vi "Module Support.vi"() -> (6 "ge_DAQManDefinitions":T1)   [LabVIEW 2012]
uses:
  Controls/DAQMan Definitions.ctl
  Custom Ctrls/ge_MeasType.ctl
  Controls/Timing Engine Support.ctl
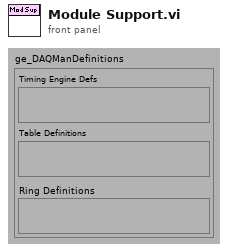
[diagram p1: front panel]
types:
  T1 = typedef "DAQMan Definitions.ctl" = cluster{"Timing Engine Defs":variant, "Table Definitions":variant, "Ring Definitions":variant}
  T2 = typedef "ge_MeasType.ctl" = enum16{"Voltage", "Frequency", "Tachometer", "Dynamic", "Thermocouple", "RTD", "Strain", "Current", "Resistance"}
  T3 = typedef "Timing Engine Support.ctl" = enum16{"HS Mod", "LS Mod", "Either"}
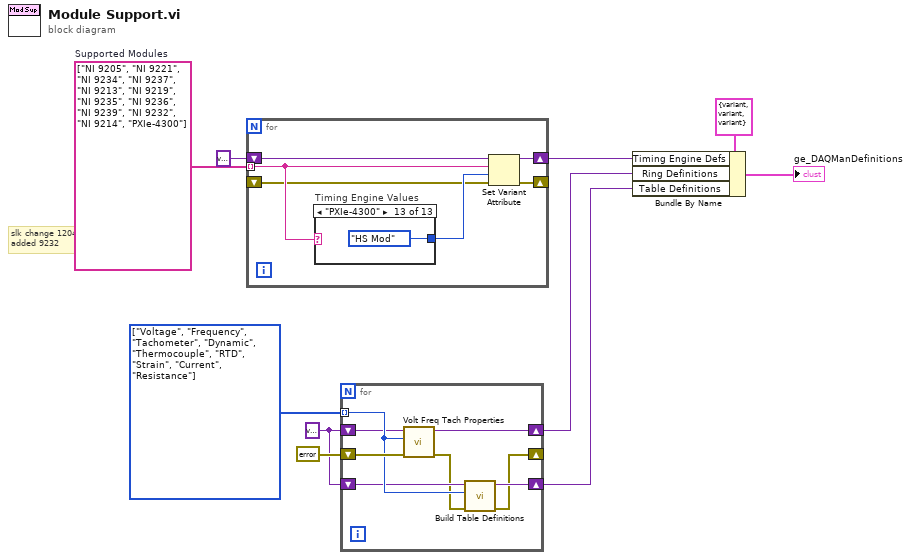
[diagram p0: block diagram]
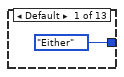
[diagram p2: hidden frame]
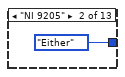
[diagram p3: hidden frame]
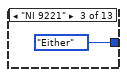
[diagram p4: hidden frame]
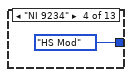
[diagram p5: hidden frame]
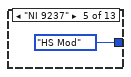
[diagram p6: hidden frame]
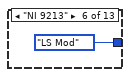
[diagram p7: hidden frame]
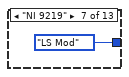
[diagram p8: hidden frame]
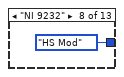
[diagram p9: hidden frame]
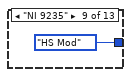
[diagram p10: hidden frame]
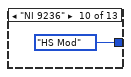
[diagram p11: hidden frame]
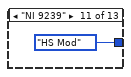
[diagram p12: hidden frame]
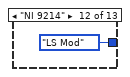
[diagram p13: hidden frame]
diagram:
  w7 = string[] ["NI 9205", "NI 9221", "NI 9234", "NI 9237", "NI 9213", "NI 9219", "NI 9235", "NI 9236", "NI 9239", "NI 9232", "NI 9214", "PXIe-4300"]  # Supported Modules
  w9 = T2[] [enum."Voltage", enum."Frequency", enum."Tachometer", enum."Dynamic", enum."Thermocouple", enum."RTD", enum."Strain", enum."Current", enum."Resistance"] items=["Voltage", "Frequency", "Tachometer", "Dynamic", "Thermocouple", "RTD", "Strain", "Current", "Resistance"]
  w8 = variant ("Rings Supported In")
  # "slk change 120423\nadded 9232"
  n1 = for {
    tunnel: w7 -> [w16] mode=indexing
    shift-right: [w13] -> w4
    shift-left: variant ("variant") -> [w14]
    shift-right: [w11] -> _
    shift-left: _ -> [w12]
    n2 = case "Timing Engine Values" shown="\"PXIe-4300\"" w16 {
      tunnel: [Timing_Engine_Support."Either" ("ValidRates") Timing_Engine_Support."Either" ("ValidRates") Timing_Engine_Support."Either" ("ValidRates") Timing_Engine_Support."HS Mod" ("ValidRates") Timing_Engine_Support."HS Mod" ("ValidRates") Timing_Engine_Support."LS Mod" ("ValidRates") Timing_Engine_Support."LS Mod" ("ValidRates") Timing_Engine_Support."HS Mod" ("ValidRates") Timing_Engine_Support."HS Mod" ("ValidRates") Timing_Engine_Support."HS Mod" ("ValidRates") Timing_Engine_Support."HS Mod" ("ValidRates") Timing_Engine_Support."LS Mod" ("ValidRates") Timing_Engine_Support."HS Mod" ("ValidRates")] -> w15
      frame Default {
      }
      frame "NI 9205" {
      }
      frame "NI 9221" {
      }
      frame "NI 9234" {
      }
      frame "NI 9237" {
      }
      frame "NI 9213" {
      }
      frame "NI 9219" {
      }
      frame "NI 9232" {
      }
      frame "NI 9235" {
      }
      frame "NI 9236" {
      }
      frame "NI 9239" {
      }
      frame "NI 9214" {
      }
      frame "PXIe-4300" {
      }
    }
    n3 = Set Variant Attribute(Variant=w14, name=w16, value=w15, error in=w12) -> (Variant out=w13:variant, error out=w11:errorcluster)  [unwired: 1 out]
  }
  n4 = for {
    shift-right: [w37] -> w3
    shift-left: w8 -> [w34]
    shift-right: [w30] -> _
    shift-left: errorcluster {"status"=FALSE, "code"=0, "source"=""} ("error out") -> [w36]
    tunnel: w9 -> [w35] mode=indexing
    shift-right: [w32] -> w1
    shift-left: w8 -> [w33]
    n5 = call "Volt Freq Tach Properties.vi"("error in"=w36, "MeasType"=w35, "Rings Supported In"=w34) -> ("error out"=w31:errorcluster, "Rings Supported Out"=w37:variant)  [unwired: 7 in]
    n6 = call "Build Table Definitions.vi"("error in (no error)"=w31, "MeasType"=w35, "Table Def In"=w33) -> ("error out"=w30:errorcluster, "Table Def Out"=w32:variant)  [unwired: 7 in]
  }
  n7 = Bundle By Name(cluster=T1 {"Timing Engine Defs"=variant, "Table Definitions"=variant, "Ring Definitions"=variant} ("ge_DAQManDefinitions"), "Timing Engine Defs"=w4, "Ring Definitions"=w3, "Table Definitions"=w1) -> (→"ge_DAQManDefinitions":T1)
